vi "DC_Link_v3.vi"(8 "error in":errorcluster, 10 "Write Channels":string="NI9264/ao0", 11 "Read Task":string="BONTS-92-DC_Link_Feedback") -> (0 "error out":errorcluster={"status"=TRUE, "code"=-200524, "source"="DC_Link_v3.vi<append>\n<B>Number of Channels in Task: </B>2\n<B>Number of Channels in Data: </B>1\n\n<B>Task Name: </B>_unnamedTask<12A>"}, 3 "DC Gain":dbl[](array[numeric]))   [LabVIEW 2021]
uses:
  <vilib>/DAQmx/write.llb/DAQmx Write (Analog 1D Wfm NChan NSamp).vi
  <vilib>/DAQmx/read.llb/DAQmx Read (Analog 1D Wfm NChan NSamp).vi
  <vilib>/DAQmx/create/channels.llb/DAQmx Create Channel (AO-Voltage-Basic).vi
  <vilib>/DAQmx/configure/timing.llb/DAQmx Timing (Sample Clock).vi
  <vilib>/measure/madcrms.llb/Basic Averaged DC-RMS for N Chan.vi
  <vilib>/DAQmx/miscellaneous.llb/DAQmx Fill In Error Info.vi
  <resource>/objmgr/daqmx.rc
  <vilib>/measure/NI_MABase.lvlib
  <vilib>/measure/NI_MAPro.lvlib
panel:
  out "Output Signal":waveform(dbl)[](graph)
  out "Input Signal":waveform(dbl)[](graph)=[{"t0"=timestamp(0 s since 1904-01-01), "dt"=0.001, "Y"=array[1000 elements]}]
  in  "Number of Samples 2":i32=1000
  in  "Sample Rate 2":dbl=1000.0
  in  "Signal 1 (5V)":tag="OnboardClock"
  out "Actual Sample Rate 2":dbl=1000.0 format="%0.2f"
  # "This test will input inverse waveforms into the DC Link -/+"
  # "And capture the DC Link Voltage, as well as the Overvoltage Fault"
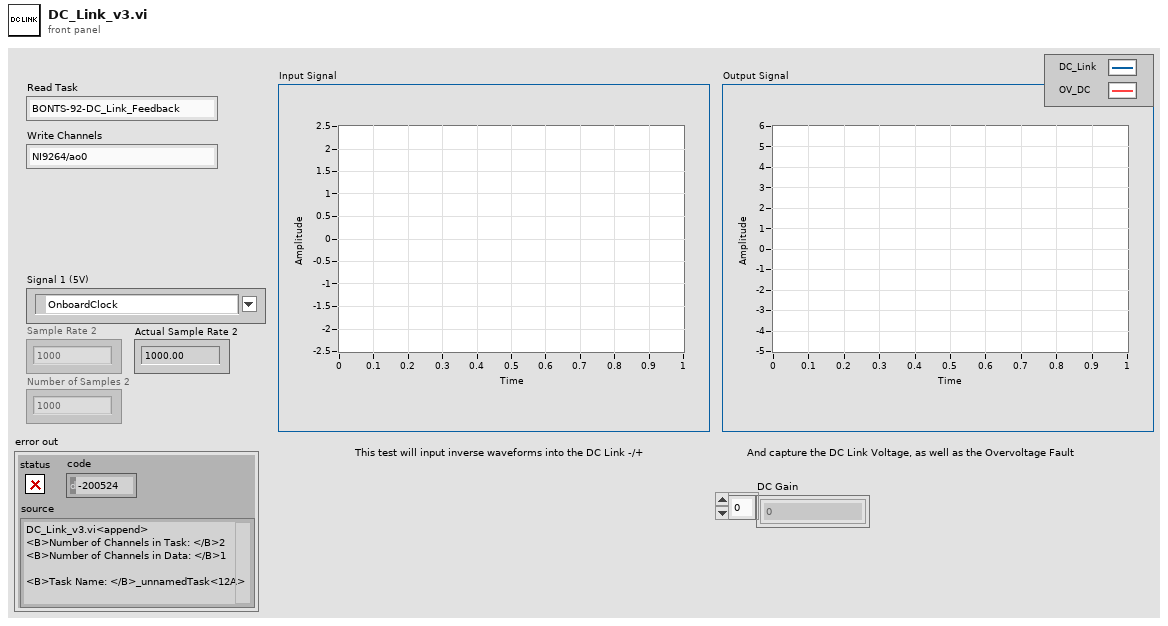
[diagram p1: front panel]
types:
  T1 = cluster{"Waveform Type":u16, "Amplitude":dbl, "Frequency":dbl}[]
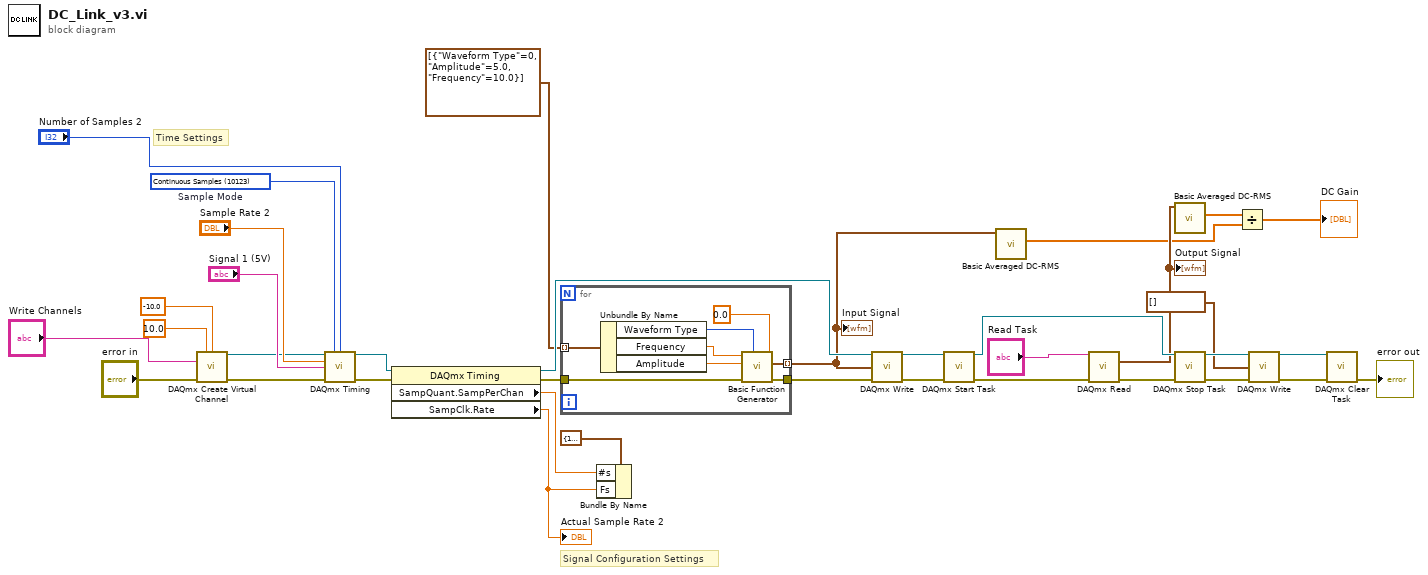
[diagram p0: block diagram]
diagram:
  w28 = 10123 items=["Finite Samples"=10178, "Continuous Samples"=10123, "Hardware Timed Single Point"=12522]  # Sample Mode
  # "Time Settings"
  # "Signal Configuration Settings"
  n1 = call-poly <vilib>:"DAQmx Create Virtual Channel.vi"("maximum value"=10.0, "minimum value"=-10.0, "physical channels"="Write Channels", "error in"="error in") -> ("task out"=w2:refnum<k21>, "error out"=w27:errorcluster)  [unwired: 10 in]
  n2 = call-poly <vilib>:"DAQmx Timing.vi"("task/channels in"=w2, "sample mode"=w28, "samples per channel"="Number of Samples 2", "rate"="Sample Rate 2", "source"="Signal 1 (5V)", "error in"=w27) -> ("task out"=w30:refnum<k21>, "error out"=w29:errorcluster)  [unwired: 8 in]
  n3 = property class="DAQmx Timing"(reference=w30, error in=w29) -> (reference out=w36:refnum<k21>, error out=w17:errorcluster, "SampQuant.SampPerChan"=w22:dbl, "SampClk.Rate"=w21:dbl)
  "Actual Sample Rate 2" <- w21
  n4 = for {
    tunnel: [w44] -> w15
    tunnel: T1 [{"Waveform Type"=0, "Amplitude"=5.0, "Frequency"=10.0}] ("Signal Input") -> [w43] mode=indexing
    tunnel: [w39] -> w3 mode=indexing
    tunnel: w17 -> [w38]
    n5 = Unbundle By Name(w43) -> ("Waveform Type"=w42:u16, "Frequency"=w41:dbl, "Amplitude"=w40:dbl)
    n6 = call <vilib>:"Basic Function Generator.vi"("offset"=0.0, "signal type"=w42, "error in (no error)"=w38, "amplitude"=w40, "frequency"=w41) -> ("error out"=w44:errorcluster, "signal out"=w39:waveform(dbl))  [unwired: 4 in, 1 out]
  }
  "Input Signal" <- w3
  n7 = Bundle By Name(cluster=cluster{"Fs":dbl, "#s":dbl} {"Fs"=1000.0, "#s"=1000.0} ("sampling info"), "#s"=w22, "Fs"=w21) -> ()  [unwired: 1 out]
  n8 = call-poly <vilib>:"DAQmx Write.vi"("task/channels in"=w36, "data"=w3, "error in"=w15) -> ("task out"=w35:refnum<k21>, "error out"=w34:errorcluster)  [unwired: 10 in, 1 out]
  n9 = call <vilib>:"DAQmx Start Task.vi"("task/channels in"=w35, "error in"=w34) -> ("task out"=w32:refnum<k21>, "error out"=w33:errorcluster)  [unwired: 12 in]
  n10 = call-poly <vilib>:"Basic Averaged DC-RMS.vi"("signals in"=w3) -> ("RMS values"=w1:dbl[])  [unwired: 7 in, 3 out]
  n11 = call-poly <vilib>:"DAQmx Read.vi"("task/channels in"="Read Task", "error in"=w33) -> ("data"=w12:waveform(dbl)[], "error out"=w31:errorcluster)  [unwired: 11 in, 1 out]
  "Output Signal" <- w12
  n12 = call-poly <vilib>:"Basic Averaged DC-RMS.vi"("signals in"=w12) -> ("RMS values"=w11:dbl[])  [unwired: 7 in, 3 out]
  n13 = call <vilib>:"DAQmx Stop Task.vi"("task/channels in"=w32, "error in"=w31) -> ("task out"=w9:refnum<k21>, "error out"=w5:errorcluster)  [unwired: 12 in]
  n14 = Divide(x=w11, y=w1) -> (x/y=→"DC Gain":dbl[])
  n15 = call-poly <vilib>:"DAQmx Write.vi"("task/channels in"=w9, "data"=waveform(dbl)[] [], "error in"=w5) -> ("task out"=w8:refnum<k21>, "error out"=w6:errorcluster)  [unwired: 10 in, 1 out]
  n16 = call <vilib>:"DAQmx Clear Task.vi"("task in"=w8, "error in"=w6) -> ("error out"=→"error out":errorcluster)  [unwired: 13 in]
